vi "tcs shm log Event Setting Versions LV.vi"(8 "error in (no error)":errorcluster, 11 "logevent_SettingVersions_Ctl":T1) -> (0 "error out":errorcluster, 2 "function return":i32, 3 "logevent_SettingVersions_Ctl out":T1)   [LabVIEW 2016, in "SALLV_tcs.lvlib"]
doc: "int tcs_shm_logEvent_SettingVersionsLV(tcs_logevent_SettingVersionsLV *logevent_SettingVersions_Ctl );"
uses:
  SALLV_tcs.lvlib
  SALLV_tcs.so
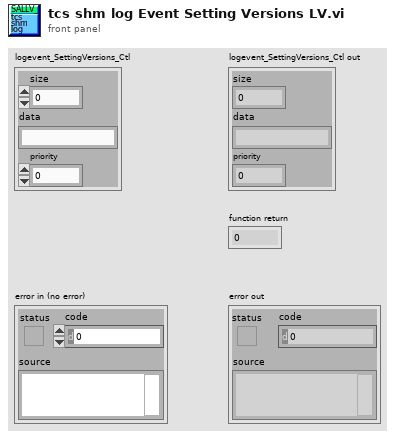
[diagram p1: front panel]
types:
  T1 = cluster{"size":i32, "data":string, "priority":i32}
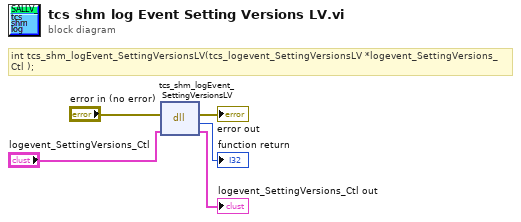
[diagram p0: block diagram]
diagram:
  # "int tcs_shm_logEvent_SettingVersionsLV(tcs_logevent_SettingVersionsLV *logevent_SettingVersions_Ctl );"
  n1 = dll-call lib="home/plotz/SALLV_tcs/SALLV_tcs.*" fn="tcs_shm_logEvent_SettingVersionsLV"(error in="error in (no error)", "logevent_SettingVersions_Ctl"="logevent_SettingVersions_Ctl") -> (error out=→"error out":errorcluster, →"function return":i32, "logevent_SettingVersions_Ctl"=→"logevent_SettingVersions_Ctl out":T1)  [unwired: 2 in, 1 out]
